vi "Create Dir.vi"(6 "error in":errorcluster, 7 "path":path) -> (2 "error out":errorcluster, 3 "path out":path)   [LabVIEW 2018]
uses:
  <vilib>/Utility/error.llb/Error Cluster From Error Code.vi
  <vilib>/ErrorRing/Error Ring.xnode
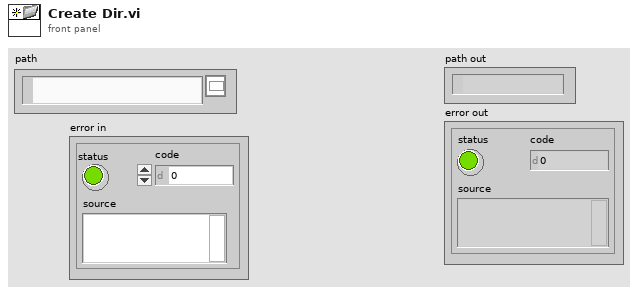
[diagram p1: front panel]
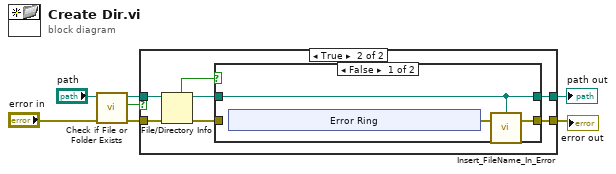
[diagram p0: block diagram]
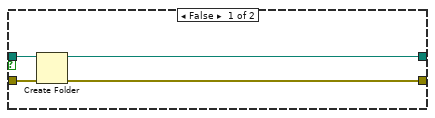
[diagram p2: hidden frame]
diagram:
  n1 = call <vilib>:"Check if File or Folder Exists.vi"("error in (no error)"="error in", "path"="path") -> ("error out"=w5:errorcluster, "file or folder exists?"=w7:bool, "dup path"=w6:path)  [unwired: 7 in]
  n2 = case shown="True" w7 {
    tunnel: w6 -> [w11 w18]
    tunnel: [w10 w15] -> w2
    tunnel: w5 -> [w9 w14]
    tunnel: [w8 w13] -> w1
    frame False {
      n3 = Create Folder(path (use dialog)=w11, error in=w9) -> (created path=w10:path, error out=w8:errorcluster)  [unwired: 1 in, 1 out]
    }
    frame True {
      n4 = File/Directory Info(path=w18, error in=w14) -> (path out=w16:path, directory=w17:bool, error out=w12:errorcluster)  [unwired: 4 out]
      n5 = case shown="False" w17 {
        tunnel: w16 -> [w19 w27]
        tunnel: [w19 w27] -> w15
        tunnel: [w20 w26] -> w13
        tunnel: w12 -> [_ w26]
        frame False {
          n6 = xnode "Error Ring"() -> ("error out"=w21:errorcluster)
          n7 = call "Insert_FileName_In_Error.vi"("error in"=w21, "Path"=w19) -> ("error out"=w20:errorcluster)  [unwired: 3 in]
        }
        frame True {
        }
      }
    }
  }
  "path out" <- w2
  "error out" <- w1
